vi "NetEventsConnect.vi"(3 "error in":errorcluster, 4 "port":u16, 5 "context in":refnum<class "zmq_context.lvclass">) -> (0 "error out":errorcluster, 1 "socket out":refnum<class "zmq_socket.lvclass">, 2 "context out":refnum<class "zmq_context.lvclass">)   [LabVIEW 2017]
uses:
  <vilib>/addons/zeromq/zmq_context.lvclass
  <vilib>/addons/zeromq/zmq_socket.lvclass
  <vilib>/addons/zeromq/socket_type.ctl
  <vilib>/addons/zeromq/socket_options.ctl
  <vilib>/addons/zeromq/zeromq.lvlib
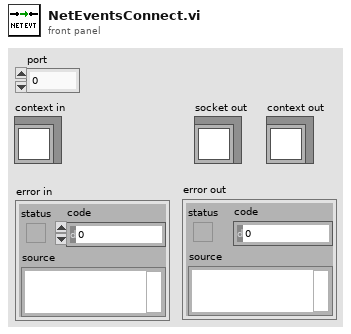
[diagram p1: front panel]
types:
  T1 = typedef "zeromq.lvlib/socket_options.ctl" = enum8{"NONE", "ZMQ_HWM", "<2>", "ZMQ_SWAP", "ZMQ_AFFINITY", "ZMQ_IDENTITY", "ZMQ_SUBSCRIBE", "ZMQ_UNSUBSCRIBE", "ZMQ_RATE", "ZMQ_RECOVERY_IVL", "ZMQ_MCAST_LOOP", "ZMQ_SNDBUF", "ZMQ_RCVBUF", "ZMQ_RCVMORE", "ZMQ_FD", "ZMQ_EVENTS", "ZMQ_TYPE", "ZMQ_LINGER", "ZMQ_RECONNECT_IVL", "ZMQ_BACKLOG", "ZMQ_RECOVERY_IVL_MSEC", "ZMQ_RECONNECT_IVL_MAX", "ZMQ_MAXMSGSIZE", "ZMQ_SNDHWM", "ZMQ_RCVHWM", "ZMQ_MULTICAST_HOPS", "<26>", "ZMQ_RCVTIMEO", "ZMQ_SNDTIMEO", "<29>", "<30>", "ZMQ_IPV4ONLY", "ZMQ_LAST_ENDPOINT", "ZMQ_ROUTER_MANDATORY", "ZMQ_TCP_KEEPALIVE", "ZMQ_TCP_KEEPALIVE_CNT", "ZMQ_TCP_KEEPALIVE_IDLE", "ZMQ_TCP_KEEPALIVE_INTVL", "ZMQ_TCP_ACCEPT_FILTER", "ZMQ_DELAY_ATTACH_ON_CONNECT", "ZMQ_XPUB_VERBOSE"}
  T2 = typedef "zeromq.lvlib/socket_type.ctl" = enum8{"ZMQ_PAIR", "ZMQ_PUB", "ZMQ_SUB", "ZMQ_REQ", "ZMQ_REP", "ZMQ_DEALER", "ZMQ_ROUTER", "ZMQ_PULL", "ZMQ_PUSH", "ZMQ_XPUB", "ZMQ_XSUB"}
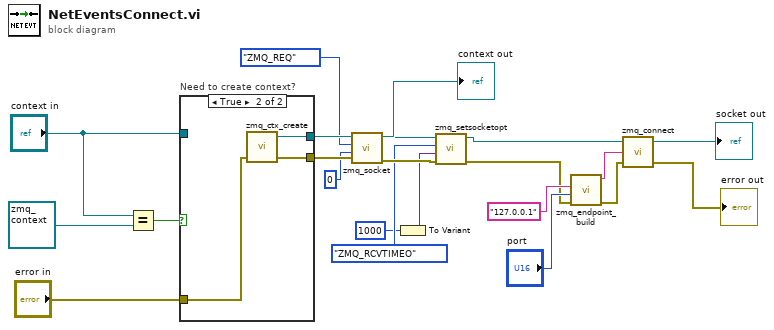
[diagram p0: block diagram]
diagram:
  n1 = Equal?(x="context in", y=refnum<class "zmq_context.lvclass"> refnum ("context in")) -> (x = y?=w21:bool)
  n2 = case "Need to create context?" shown="True" w21 {
    tunnel: [w24 w27] -> w18
    tunnel: [w23 w26] -> w17
    tunnel: "context in" -> [w24 _]
    tunnel: "error in" -> [w23 w25]
    frame False {
    }
    frame True {
      n3 = call <vilib>:"zmq_ctx_create.vi"("error in"=w25) -> ("error out"=w26:errorcluster, "context out"=w27:refnum<class "zmq_context.lvclass">)  [unwired: 3 in]
    }
  }
  n4 = call <vilib>:"zmq_socket.vi"("error in"=w17, "linger (ms)"=0, "socket type"=socket_type."ZMQ_REQ", "context in"=w18) -> ("error out"=w6:errorcluster, "socket out"=w7:refnum<class "zmq_socket.lvclass">, "context out"=→"context out":refnum<class "zmq_context.lvclass">)  [unwired: 1 in]
  n5 = To Variant(anything=1000) -> (Variant=w1:variant)
  n6 = call <vilib>:"zmq_setsocketopt.vi"("error in"=w6, "value"=w1, "option"=socket_options."ZMQ_RCVTIMEO", "socket in"=w7) -> ("error out"=w5:errorcluster, "socket out"=w4:refnum<class "zmq_socket.lvclass">)  [unwired: 2 in]
  n7 = call <vilib>:"zmq_endpoint_build.vi"("error in"=w5, "port"="port", "address"="127.0.0.1") -> ("error out"=w11:errorcluster, "endpoint"=w12:string)  [unwired: 2 in, 1 out]
  n8 = call <vilib>:"zmq_connect.vi"("error in"=w11, "endpoint"=w12, "socket in"=w4) -> ("error out"=→"error out":errorcluster, "socket out"=→"socket out":refnum<class "zmq_socket.lvclass">)  [unwired: 1 in]
